vi "Convert Bertec CSV into dynamic data type.vi"(0 "selected path":path, 1 "Input Datafile Separator":enum32{"CSV", "TSV"}(radio)) -> (2 "Dynamic Data Type":dynamicdata(waveform))   [LabVIEW 2016]
uses:
  <vilib>/Utility/file.llb/Read Delimited Spreadsheet (DBL).vi
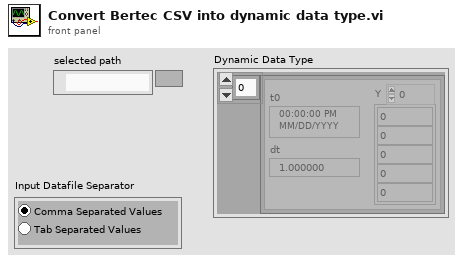
[diagram p1: front panel]
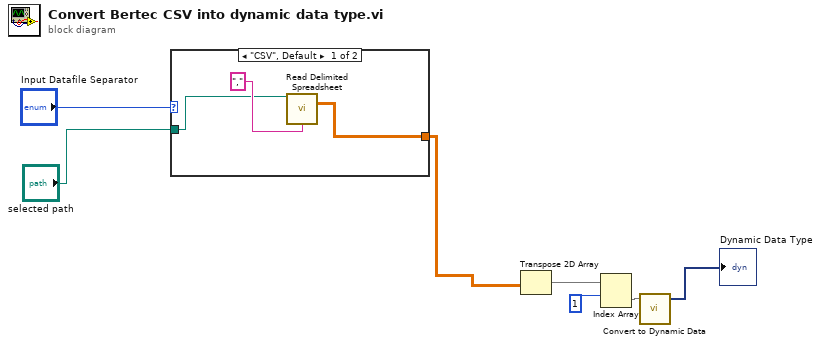
[diagram p0: block diagram]
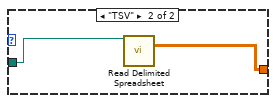
[diagram p2: hidden frame]
diagram:
  n1 = case shown="\"CSV\", Default" "Input Datafile Separator" {
    tunnel: "selected path" -> [w9 w12]
    tunnel: [w8 w11] -> w1
    frame "CSV", Default {
      n2 = call-poly <vilib>:"Read Delimited Spreadsheet.vi"("file path (dialog if empty)"=w9, "delimiter (\\t)"="," ("delimiter")) -> ("all rows"=w8:dbl[][])  [unwired: 8 in, 5 out]
    }
    frame "TSV" {
      n3 = call-poly <vilib>:"Read Delimited Spreadsheet.vi"("file path (dialog if empty)"=w12) -> ("all rows"=w11:dbl[][])  [unwired: 9 in, 5 out]
    }
  }
  n4 = Transpose 2D Array(2D array=w1) -> (transposed array=w5:dbl[][])
  n5 = Index Array(array=w5, index (row)=1) -> (element=w6:dbl[])  [unwired: 1 in]
  n6 = call "Convert to Dynamic Data"("Array"=w6) -> ("Dynamic Data Type"=→"Dynamic Data Type":dynamicdata)  [unwired: 3 in]
